vi "Get Port Number.vi"(8 "error in":errorcluster, 11 "port ref in":T1 format="%.0x") -> (0 "error out":errorcluster, 2 "port number":u16, 3 "port ref out":T1 format="%.0x", 4 "found?":bool)   [LabVIEW 2020, in "Communication Bus Template Scripting.lvlib"]
uses:
  Communication Bus Template Scripting.lvlib
  <vilib>/NI VeriStand/Custom Device API/Custom Device Item Ref.ctl
  Constants.vi
  <vilib>/NI VeriStand/Custom Device API/Get Item Property (U16).vi
  <vilib>/NI VeriStand/Custom Device API/Custom Device API.lvlib
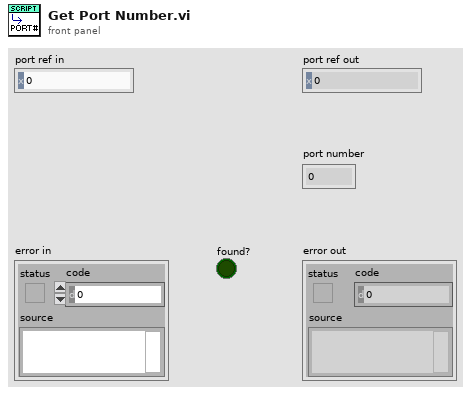
[diagram p1: front panel]
types:
  T1 = typedef "Custom Device API.lvlib/Custom Device Item Ref.ctl" = u64
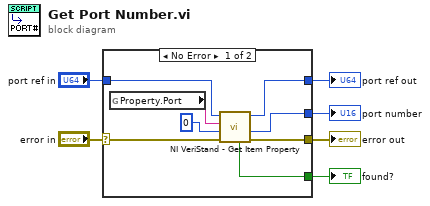
[diagram p0: block diagram]
diagram:
  n1 = case shown="No Error" "error in" {
    selector: "error in" -> [w13 w15]
    tunnel: "port ref in" -> [w11 w16]
    tunnel: [w10 w15] -> w4
    tunnel: [w9 _] -> w3
    tunnel: [w8 w16] -> w2
    tunnel: [w7 _] -> w1
    frame No Error {
      n2 = global read "Constants.vi" "Property.Port"() -> (w14:string)
      n3 = call-poly <vilib>:"NI VeriStand - Get Item Property.vi"("error in (no error)"=w13, "Default Value"=u16 0, "Property Name"=w14, "Item Ref in"=w11) -> ("error out"=w10:errorcluster, "Value"=w9:u16, "Item Ref out"=w8:T1, "Found?"=w7:bool)  [unwired: 4 in]
    }
    frame Error {
    }
  }
  "error out" <- w4
  "port number" <- w3
  "port ref out" <- w2
  "found?" <- w1
